vi "Max Block Count.vi"   [LabVIEW 2017, in "DSF Core.lvlib"]
uses:
  DSF Core.lvlib
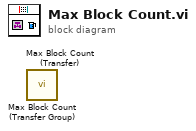
[diagram p0: block diagram]
diagram:
  n1 = call "Max Block Count (Transfer Group).vi"() -> ()  [unwired: 9 in, 3 out]
  n2 = call "Max Block Count (Transfer).vi"() -> ()  [unwired: 9 in, 3 out]
